vi "cmd_approach.vi"(8 "error in (no error)":errorcluster, 11 "JSON":string) -> (0 "error out":errorcluster)   [LabVIEW 2021]
doc: "Perform an approach using the coarse approach mechanism with sawtooth wave signals. \n \n Before calling this command, an approaced condition should be set \n by set_threshold command.\n\n :param sleep: Specifies the delay between z2 motion and z motion\n :param avg: Specifies the average count for z\n :param dz: Specifies the change of z\n :param zstart: Specifies the start position of z\n :param zend: Specifies the end position of z\n :param z2ch: Specifies the z2 channel for sawtooth wave\n :param avg2: Specifies the average count for z2\n :param dz2: Specifies the change of z2\n :param z2start: Specifies the start position of z2\n :param z2end: Specifies the end position of z2"
uses:
  fpga/fpga_dtype_scan_config.ctl
  fpga/fpga_dtype_sgl_8ch.ctl
  fpga/fpga_dtype_index.ctl
  core/host_global_vars.vi
panel:
  in  "args":T1
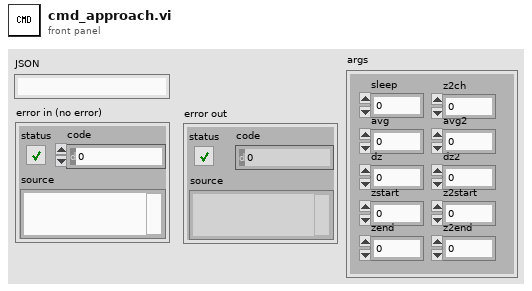
[diagram p1: front panel]
types:
  T1 = cluster{"sleep":i32, "avg":i32, "dz":sgl, "zstart":sgl, "zend":sgl, "z2ch":i32, "avg2":i32, "dz2":sgl, "z2start":sgl, "z2end":sgl}
  T2 = typedef "fpga_dtype_sgl_8ch.ctl" = cluster{"ch 0":sgl, "ch 1":sgl, "ch 2":sgl, "ch 3":sgl, "ch 4":sgl, "ch 5":sgl, "ch 6":sgl, "ch 7":sgl}
  T3 = cluster{"target[0]":sgl, "target[1]":sgl, "target[2]":sgl, "target[3]":sgl, "target[4]":sgl, "target[5]":sgl, "target[6]":sgl, "target[7]":sgl}
  T4 = typedef "fpga_dtype_index.ctl" = cluster{"page":i16, "2nd":i16, "1st":i16}
  T5 = typedef "fpga_dtype_scan_config.ctl" = cluster{"data points":i16, "average counts":i16, "delta per point":T2, "bidirectional scan":bool, "auto reversal":bool}
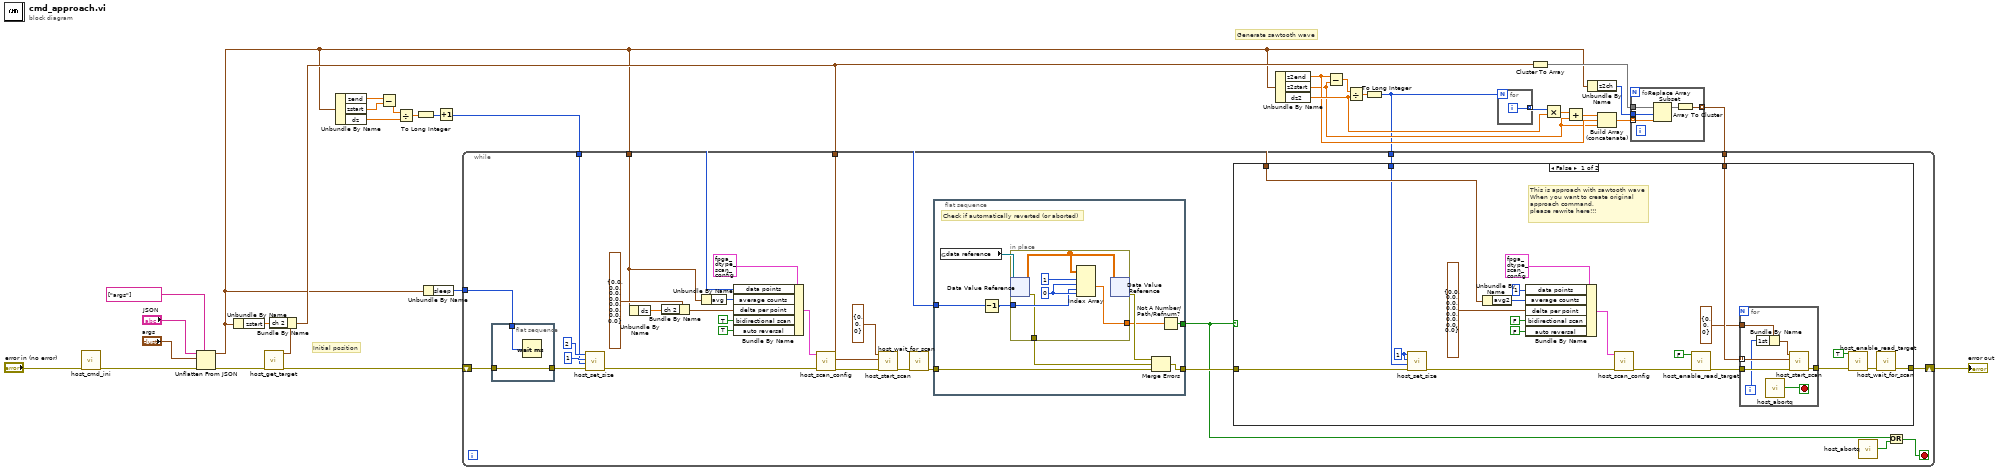
[diagram p0: block diagram]
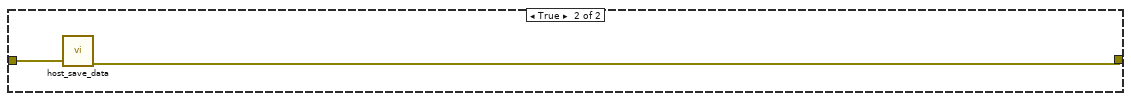
[diagram p2: hidden frame]
diagram:
  # "Initial position"
  # "Generate sawtooth wave"
  n1 = call "host_cmd_ini.vi"("error in (no error)"="error in (no error)") -> ("error out"=w30:errorcluster)  [unwired: 10 in]
  n2 = Unflatten From JSON(path=string[] ["args"], JSON string="JSON", type and defaults="args", error in (no error)=w30) -> (value=w3:T1, error out=w26:errorcluster)  [unwired: 3 in]
  n3 = Unbundle By Name(w3) -> ("zstart"=w18:sgl)
  n4 = call "host_get_target.vi"("error in"=w26) -> ("error out"=w1:errorcluster, "target"=w19:T2)  [unwired: 9 in]
  n5 = Bundle By Name(cluster=w19, "ch 2"=w18) -> (w7:T2)
  n6 = Unbundle By Name(w3) -> ("zend"=w14:sgl, "zstart"=w13:sgl, "dz"=w11:sgl)
  n7 = Subtract(x=w14, y=w13) -> (x-y=w12:sgl)
  n8 = Divide(x=w12, y=w11) -> (x/y=w10:sgl)
  n9 = To Long Integer(number=w10) -> (32bit integer=w9:i32)
  n10 = Unbundle By Name(w3) -> ("sleep"=w2:i32)
  n11 = Increment(x=w9) -> (x+1=w6:i32)
  n12 = Unbundle By Name(w3) -> ("z2end"=w21:sgl, "z2start"=w20:sgl, "dz2"=w23:sgl)
  n13 = Subtract(x=w21, y=w20) -> (x-y=w25:sgl)
  n14 = Divide(x=w25, y=w23) -> (x/y=w28:sgl)
  n15 = To Long Integer(number=w28) -> (32bit integer=w5:i32)
  n16 = for {
    N: w5 -> [_]
    tunnel: [w34] -> w27 mode=indexing
    i -> [w34]
  }
  n17 = Cluster To Array(cluster=w7) -> (array=w16:sgl[])
  n18 = Multiply(x=w27, y=w23) -> (x*y=w24:sgl[])
  n19 = Add(x=w24, y=w20) -> (x+y=w22:sgl[])
  n20 = Unbundle By Name(w3) -> ("z2ch"=w15:i32)
  n21 = Build Array (concatenate)(w22, w21, w20) -> (w17:sgl[])
  n22 = for {
    tunnel: w17 -> [w38] mode=indexing
    tunnel: w16 -> [w39]
    tunnel: w15 -> [w37]
    tunnel: [w35] -> w8 mode=indexing
    n23 = Replace Array Subset(array=w39, new element=w38, index=w37) -> (w36:sgl[])
    n24 = Array To Cluster(array=w36) -> (cluster=w35:T3)
  }
  n25 = while {
    tunnel: w8 -> [w65]
    tunnel: w7 -> [w64]
    tunnel: w6 -> [w51]
    tunnel: w5 -> [w48]
    tunnel: w3 -> [w46]
    tunnel: w2 -> [w45]
    shift-right: [w47] -> w4
    shift-left: w1 -> [w43]
    stop <- w40 stop-if-true
    n26 = flat-sequence {
      tunnel: w45 -> [w69]
      tunnel: [w68] -> w44
      tunnel: w43 -> [w68]
      frame #0 {
        n27 = Wait (ms)(milliseconds to wait=w69) -> ()  [unwired: 1 out]
      }
    }
    n28 = call "host_set_size.vi"("error in (no error)"=w44, "fast"=w51, "slow"=1, "page"=2) -> ("error out"=w52:errorcluster)  [unwired: 7 in]
    n29 = Unbundle By Name(w46) -> ("dz"=w60:sgl)
    n30 = Bundle By Name(cluster=T2 {"ch 0"=0.0, "ch 1"=0.0, "ch 2"=0.0, "ch 3"=0.0, "ch 4"=0.0, "ch 5"=0.0, "ch 6"=0.0, "ch 7"=0.0} ("delta per point"), "ch 2"=w60) -> (w61:T2)
    n31 = Unbundle By Name(w46) -> ("avg"=w59:i32)
    n32 = Bundle By Name(cluster=T5 {"data points"=0, "average counts"=0, "delta per point"={"ch 0"=0.0, "ch 1"=0.0, "ch 2"=0.0, "ch 3"=0.0, "ch 4"=0.0, "ch 5"=0.0, "ch 6"=0.0, "ch 7"=0.0}, "bidirectional scan"=FALSE, "auto reversal"=FALSE} ("scan config"), "data points"=w51, "average counts"=w59, "delta per point"=w61, "bidirectional scan"=TRUE, "auto reversal"=TRUE) -> (w58:T5)
    n33 = call "host_scan_config.vi"("error in"=w52, "scan config"=w58) -> ("error out"=w62:errorcluster)  [unwired: 9 in]
    n34 = call "host_start_scan.vi"("error in"=w62, "initial positions"=w64, "index offset"=T4 {"page"=0, "2nd"=0, "1st"=0}) -> ("error out"=w63:errorcluster)  [unwired: 6 in, 2 out]
    n35 = call "host_wait_for_scan.vi"("error in (no error)"=w63) -> ("error out"=w50:errorcluster)  [unwired: 10 in]
    n36 = flat-sequence {
      tunnel: w51 -> [w106]
      tunnel: w50 -> [w104]
      tunnel: [w100] -> w41
      tunnel: [w102] -> w49
      frame #0 {
        # "Check if automatically reverted (or aborted)"
        n37 = global read "host_global_vars.vi" "data reference"() -> (w108:refnum<data-value>)
        n38 = Decrement(x=w106) -> (x-1=w107:i32)
        n39 = in-place {
          in-place-border: w107 -> [w111]
          in-place-border: [w110] -> w103
          in-place-border: [w109] -> w101
          w113 = 0 ("index (vol)")
          n40 = in-place-dvr #1(w108) -> (w112:sgl[][][][], w110:errorcluster)
          n41 = Index Array(array=w112, index (dim 0)=1 ("index (vol)"), index (dim 1)=w113, index (dim 2)=w111, index (dim 3)=w113) -> (element=w109:sgl)
          n42 = in-place-dvr #1(w112) -> (w105:errorcluster)  [unwired: 1 out]
        }
        n43 = Merge Errors(w105, w103, w104) -> (w102:errorcluster)
        n44 = Not A Number/Path/Refnum?(number/path/refnum=w101) -> (NaN/Path/Refnum?=w100:bool)
      }
    }
    n45 = case shown="False" w41 {
      tunnel: w65 -> [w90 _]
      tunnel: w46 -> [w74 _]
      tunnel: w49 -> [w73 w99]
      tunnel: w48 -> [w72 _]
      tunnel: [w70 w98] -> w47
      frame False {
        w71 = 1 ("page")
        # "This is approach with sawtooth wave\nWhen you want to create original \napproach command,\nplease rewrite here!!!"
        n46 = call "host_set_size.vi"("error in (no error)"=w73, "fast"=w72, "slow"=w71, "page"=w71) -> ("error out"=w75:errorcluster)  [unwired: 7 in]
        n47 = Unbundle By Name(w74) -> ("avg2"=w86:i32)
        n48 = Bundle By Name(cluster=T5 {"data points"=0, "average counts"=0, "delta per point"={"ch 0"=0.0, "ch 1"=0.0, "ch 2"=0.0, "ch 3"=0.0, "ch 4"=0.0, "ch 5"=0.0, "ch 6"=0.0, "ch 7"=0.0}, "bidirectional scan"=FALSE, "auto reversal"=FALSE} ("scan config"), "data points"=i16 1, "average counts"=w86, "delta per point"=T2 {"ch 0"=0.0, "ch 1"=0.0, "ch 2"=0.0, "ch 3"=0.0, "ch 4"=0.0, "ch 5"=0.0, "ch 6"=0.0, "ch 7"=0.0}, "bidirectional scan"=FALSE, "auto reversal"=FALSE) -> (w82:T5)
        n49 = call "host_scan_config.vi"("error in"=w75, "scan config"=w82) -> ("error out"=w81:errorcluster)  [unwired: 9 in]
        n50 = call "host_enable_read_target.vi"("error in"=w81, "enable read target?"=FALSE ("hold")) -> ("error out"=w80:errorcluster)  [unwired: 9 in]
        n51 = for {
          tunnel: w80 -> [w97]
          tunnel: T4 {"page"=0, "2nd"=0, "1st"=0} ("index offset") -> [w93]
          tunnel: w90 -> [w96] mode=indexing
          tunnel: [w94] -> w77
          i -> [w91]
          stop <- w95 stop-if-true
          n52 = Bundle By Name(cluster=w93, "1st"=w91) -> (w92:T4)
          n53 = call "host_abortq.vi"() -> ("abort"=w95:bool)  [unwired: 1 in]
          n54 = call "host_start_scan.vi"("error in"=w97, "initial positions"=w96, "index offset"=w92) -> ("error out"=w94:errorcluster)  [unwired: 6 in, 2 out]
        }
        n55 = call "host_enable_read_target.vi"("error in"=w77, "enable read target?"=TRUE ("hold")) -> ("error out"=w76:errorcluster)  [unwired: 9 in]
        n56 = call "host_wait_for_scan.vi"("error in (no error)"=w76) -> ("error out"=w70:errorcluster)  [unwired: 10 in]
      }
      frame True {
        n57 = call "host_save_data.vi"("error in"=w99) -> ("error out"=w98:errorcluster)  [unwired: 10 in]
      }
    }
    n58 = call "host_abortq.vi"() -> ("abort"=w42:bool)  [unwired: 1 in]
    n59 = Or(x=w41, y=w42) -> (x .or. y?=w40:bool)
  }
  "error out" <- w4
